vi "BuildSequence.vi"(1 "Connections":string[](array[string])) -> (0 "Sequence":string[](array[string]))   [LabVIEW 2015]
panel:
  in  "Initial Crosshair":string="00 | 01"
  out "Target Crosshair":string
  out "Current Crosshair":string="00 | 01"
  out "Target Device":string
  out "Current Device":string="00"
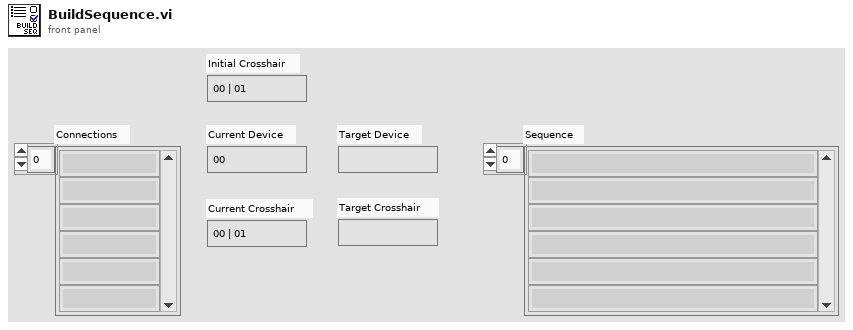
[diagram p1: front panel]
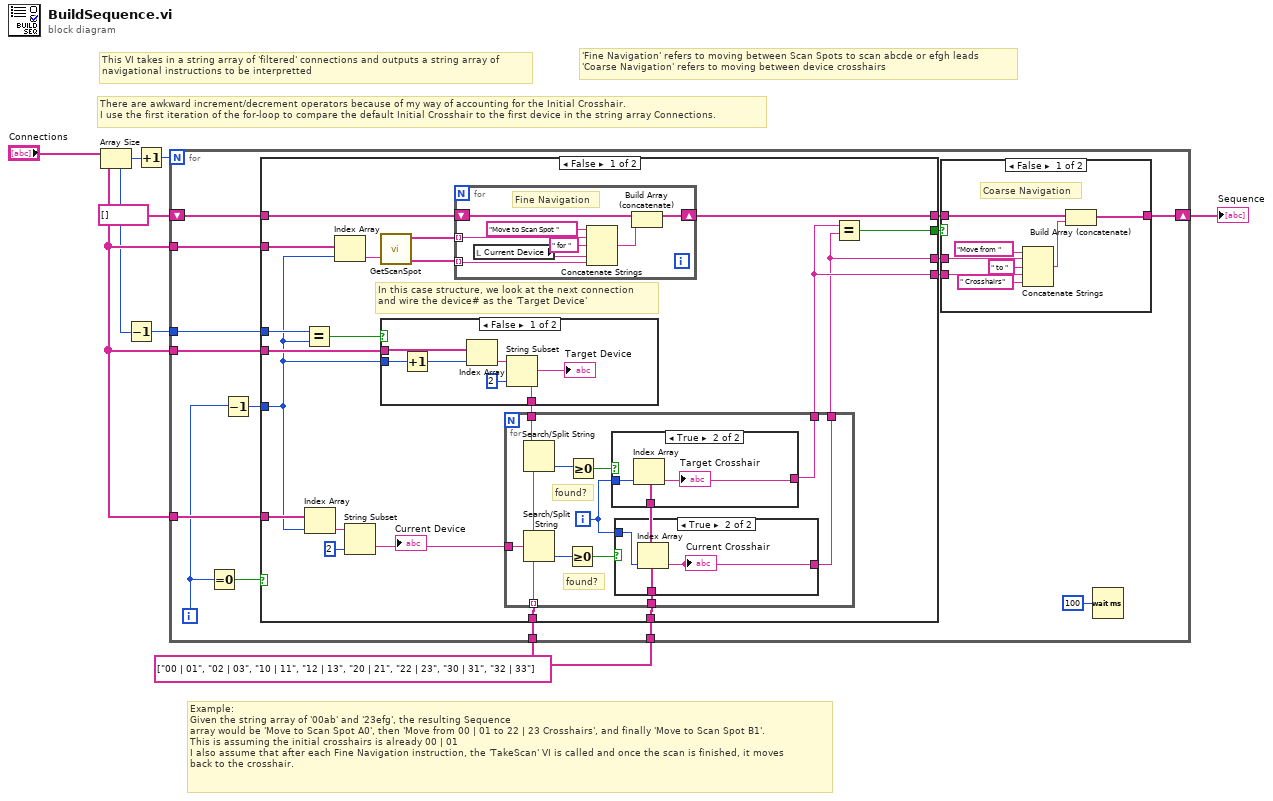
[diagram p0: block diagram]
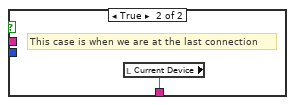
[diagram p2: hidden frame]
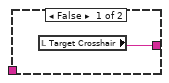
[diagram p3: hidden frame]
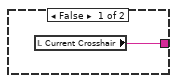
[diagram p4: hidden frame]
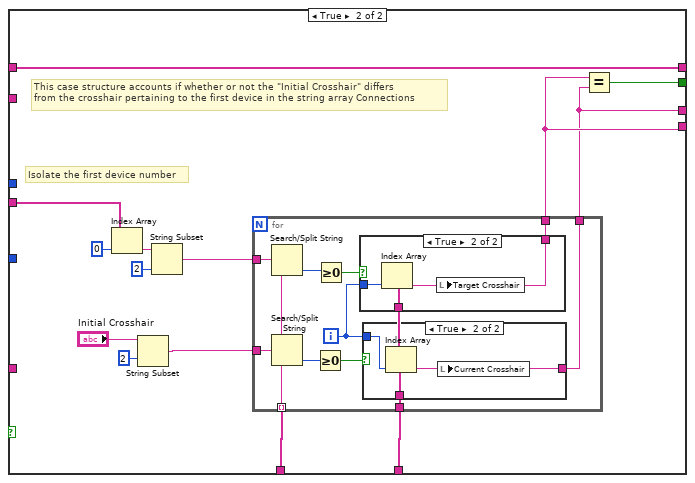
[diagram p5: hidden frame]
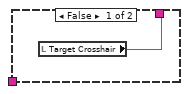
[diagram p6: hidden frame]
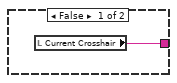
[diagram p7: hidden frame]
diagram:
  w3 = string[] ["00 | 01", "02 | 03", "10 | 11", "12 | 13", "20 | 21", "22 | 23", "30 | 31", "32 | 33"]
  # "'Fine Navigation' refers to moving between Scan Spots to scan abcde or efgh leads\n'Coarse Navigation' refers to moving between device crosshairs"
  # "Example: \nGiven the string array of '00ab' and '23efg', the resulting Sequence\narray would be 'Move to Scan Spot A0', then 'Move from 00 | 01 to 22 | 23 Crosshairs', and finally 'Move to Scan Spot B1'.\nThis is assuming the initial crosshairs is already 00 | 01\nI also assume that after each Fine Navigation instruction, the 'TakeScan' VI is called and once the scan is finished, it moves\nback to the crosshair."
  # "This VI takes in a string array of 'filtered' connections and outputs a string array of\nnavigational instructions to be interpretted"
  # "There are awkward increment/decrement operators because of my way of accounting for the Initial Crosshair. \nI use the first iteration of the for-loop to compare the default Initial Crosshair to the first device in the string array Connections."
  n1 = Array Size(array="Connections") -> (size(s)=w1:i32)
  n2 = Decrement(x=w1) -> (x-1=w7:i32)
  n3 = Increment(x=w1) -> (x+1=w2:i32)
  n4 = for {
    N: w2 -> [_]
    tunnel: w3 -> [w22]
    tunnel: w7 -> [w23]
    shift-right: [w19] -> w6
    shift-left: string[] [] -> [w16]
    tunnel: "Connections" -> [w18]
    tunnel: "Connections" -> [w17]
    tunnel: "Connections" -> [w12]
    tunnel: w3 -> [w11]
    i -> [w9]
    n5 = Equal To 0?(x=w9) -> (x = 0?=w10:bool)
    n6 = Decrement(x=w9) -> (x-1=w8:i32)
    n7 = case shown="False" w10 {
      tunnel: w23 -> [w43 _]
      tunnel: w22 -> [w42 w88]
      tunnel: [w40 w80] -> w20
      tunnel: w18 -> [w39 w83]
      tunnel: w17 -> [w38 _]
      tunnel: w16 -> [w37 w81]
      tunnel: [w36 w81] -> w15
      tunnel: [w35 w79] -> w14
      tunnel: [w34 w78] -> w13
      tunnel: w12 -> [w27 _]
      tunnel: w11 -> [w25 w87]
      tunnel: w8 -> [w24 _]
      frame False {
        # "In this case structure, we look at the next connection \nand wire the device# as the 'Target Device'"
        n8 = Equal?(x=w43, y=w24) -> (x = y?=w33:bool)
        n9 = Index Array(array=w27, index=w24) -> (element=w28:string)
        n10 = Index Array(array=w38, index=w24) -> (element=w32:string)
        n11 = String Subset(string=w28, length (rest)=2 ("length (rest)")) -> (substring=w26:string)  [unwired: 1 in]
        "Current Device" <- w26
        n12 = call "GetScanSpot.vi"("Device to Scan"=w32) -> ("Scan Spot"=w31:string[], "Scanned Leads"=w30:string[])
        n13 = case shown="False" w33 {
          tunnel: w39 -> [w49 _]
          tunnel: [w46 w50] -> w41
          tunnel: w24 -> [w44 _]
          frame False {
            n14 = Increment(x=w44) -> (x+1=w45:i32)
            n15 = Index Array(array=w49, index=w45) -> (element=w47:string)
            n16 = String Subset(string=w47, length (rest)=2 ("length (rest)")) -> (substring=w46:string)  [unwired: 1 in]
            "Target Device" <- w46
          }
          frame True {
            # "This case is when we are at the last connection"
            n17 = local read "Current Device"() -> (w50:string)
          }
        }
        n18 = for {
          shift-right: [w58] -> w36
          shift-left: w37 -> [w56]
          tunnel: w31 -> [w54] mode=indexing
          tunnel: w30 -> [w51] mode=indexing
          # "Fine Navigation"
          n19 = local read "Current Device"() -> (w52:string)
          n20 = Concatenate Strings("Move to Scan Spot " ("string"), w54, " for " ("string"), w52, w51) -> (w55:string)
          n21 = Build Array (concatenate)(w56, w55) -> (w58:string[])
        }
        n22 = for {
          tunnel: w42 -> [w60] mode=indexing
          tunnel: w25 -> [w65]
          tunnel: w41 -> [w64]
          tunnel: [w62] -> w35
          tunnel: [w61] -> w34
          tunnel: w26 -> [w59]
          i -> [w63]
          # "found?"
          # "found?"
          n23 = Search/Split String(string=w60, search string/char (-)=w64) -> (offset of match=w66:i32)  [unwired: 1 in, 2 out]
          n24 = Search/Split String(string=w60, search string/char (-)=w59) -> (offset of match=w68:i32)  [unwired: 1 in, 2 out]
          n25 = Greater Or Equal To 0?(x=w68) -> (x >= 0?=w69:bool)
          n26 = Greater Or Equal To 0?(x=w66) -> (x >= 0?=w67:bool)
          n27 = case shown="True" w67 {
            tunnel: w63 -> [_ w72]
            tunnel: w65 -> [_ w73]
            tunnel: [w70 w71] -> w62
            frame False {
              n28 = local read "Target Crosshair"() -> (w70:string)
            }
            frame True {
              n29 = Index Array(array=w73, index=w72) -> (element=w71:string)
              "Target Crosshair" <- w71
            }
          }
          n30 = case shown="True" w69 {
            tunnel: w65 -> [_ w77]
            tunnel: w63 -> [_ w76]
            tunnel: [w74 w75] -> w61
            frame False {
              n31 = local read "Current Crosshair"() -> (w74:string)
            }
            frame True {
              n32 = Index Array(array=w77, index=w76) -> (element=w75:string)
              "Current Crosshair" <- w75
            }
          }
        }
        n33 = Equal?(x=w35, y=w34) -> (x = y?=w40:bool)
      }
      frame True {
        # "This case structure accounts if whether or not the \"Initial Crosshair\" differs\nfrom the crosshair pertaining to the first device in the string array Connections"
        # "Isolate the first device number"
        n34 = Index Array(array=w83, index=0) -> (element=w85:string)
        n35 = String Subset(string="Initial Crosshair", length (rest)=2 ("length (rest)")) -> (substring=w89:string)  [unwired: 1 in]
        n36 = String Subset(string=w85, length (rest)=2 ("length (rest)")) -> (substring=w84:string)  [unwired: 1 in]
        n37 = for {
          tunnel: w88 -> [w94] mode=indexing
          tunnel: w87 -> [w98]
          tunnel: [w96] -> w79
          tunnel: [w95] -> w78
          tunnel: w89 -> [w93]
          tunnel: w84 -> [w92]
          i -> [w97]
          n38 = Search/Split String(string=w94, search string/char (-)=w92) -> (offset of match=w99:i32)  [unwired: 1 in, 2 out]
          n39 = Search/Split String(string=w94, search string/char (-)=w93) -> (offset of match=w101:i32)  [unwired: 1 in, 2 out]
          n40 = Greater Or Equal To 0?(x=w101) -> (x >= 0?=w102:bool)
          n41 = Greater Or Equal To 0?(x=w99) -> (x >= 0?=w100:bool)
          n42 = case shown="True" w100 {
            tunnel: w97 -> [_ w105]
            tunnel: w98 -> [_ w106]
            tunnel: [w103 w104] -> w96
            frame False {
              n43 = local read "Target Crosshair"() -> (w103:string)
            }
            frame True {
              n44 = Index Array(array=w106, index=w105) -> (element=w104:string)
              n45 = local write "Target Crosshair"(w104) -> ()
            }
          }
          n46 = case shown="True" w102 {
            tunnel: w98 -> [_ w110]
            tunnel: w97 -> [_ w109]
            tunnel: [w107 w108] -> w95
            frame False {
              n47 = local read "Current Crosshair"() -> (w107:string)
            }
            frame True {
              n48 = Index Array(array=w110, index=w109) -> (element=w108:string)
              n49 = local write "Current Crosshair"(w108) -> ()
            }
          }
        }
        n50 = Equal?(x=w79, y=w78) -> (x = y?=w80:bool)
      }
    }
    n51 = case shown="False" w20 {
      tunnel: [w112 w119] -> w19
      tunnel: w13 -> [w117 _]
      tunnel: w14 -> [w115 _]
      tunnel: w15 -> [w114 w119]
      frame False {
        # "Coarse Navigation"
        n52 = Concatenate Strings("Move from " ("string"), w117, " to " ("string"), w115, " Crosshairs" ("string")) -> (w113:string)
        n53 = Build Array (concatenate)(w114, w113) -> (w112:string[])
      }
      frame True {
        # "If Current and Target Crosshairs\nare equal, then no need for \nCoarse Navigation"
      }
    }
    n54 = Wait (ms)(milliseconds to wait=u32 100) -> ()  [unwired: 1 out]
  }
  "Sequence" <- w6
